vi "维持时间参数检查.vi"(7 "队列输入":refnum<queue>, 8 "NewVal输入":T1 {"时序参数"."nplc" min=0.001; "测试参数"."极限电流(mA)" min=0.0 max=3000.0; "测试参数"."读取电压(V)" min=0.0 max=40.0}, 11 "错误输入（无错误）":errorcluster) -> (0 "NewVal输出":T1 {"时序参数"."nplc" min=0.001; "测试参数"."极限电流(mA)" min=0.0 max=3000.0; "测试参数"."读取电压(V)" min=0.0 max=40.0}, 3 "错误输出":errorcluster)   [LabVIEW 2021]
uses:
  QueueLib/QueueLib.lvlib
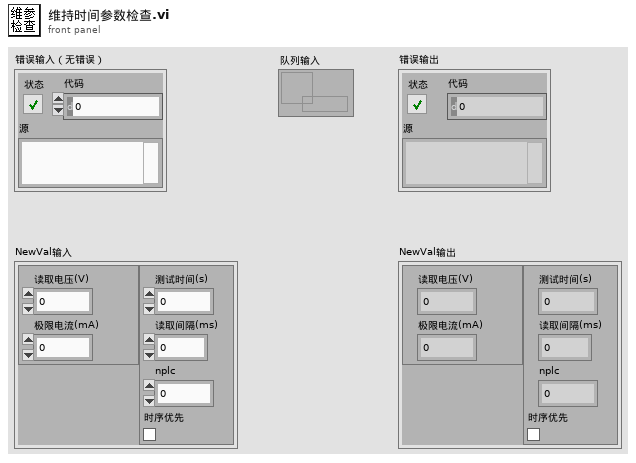
[diagram p1: front panel]
types:
  T1 = typedef "维持时间.ctl" = cluster{"测试参数":cluster{"读取电压(V)":dbl, "极限电流(mA)":dbl}, "时序参数":cluster{"测试时间(s)":dbl, "读取间隔(ms)":dbl, "nplc":dbl, "时序优先":bool}}
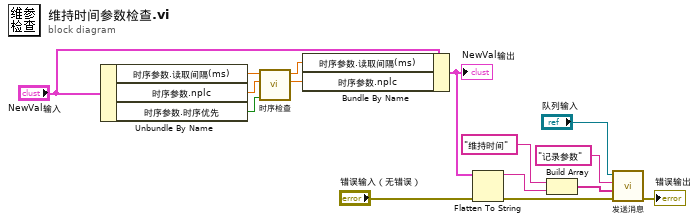
[diagram p0: block diagram]
diagram:
  n1 = Unbundle By Name("NewVal输入") -> ("时序参数.读取间隔(ms)"=w1:dbl, "时序参数.nplc"=w2:dbl, "时序参数.时序优先"=w3:bool)
  n2 = call "时序检查.vi"("时序优先"=w3, "nplc"=w2, "测量间隔"=w1) -> ("nplc输出"=w5:dbl, "测量间隔输出"=w4:dbl)  [unwired: 7 in]
  n3 = Bundle By Name(cluster="NewVal输入", "时序参数.读取间隔(ms)"=w4, "时序参数.nplc"=w5) -> (w15:T1)
  "NewVal输出" <- w15
  n4 = Flatten To String(anything=w15, error in (no error)="错误输入（无错误）") -> (data string=w8:string, error out=w6:errorcluster)  [unwired: 2 in, 1 out]
  n5 = Build Array("维持时间" ("元素"), w8) -> (w10:string[])
  n6 = call-poly "发送消息.vi"("错误输入（无错误）"=w6, "数据"=w10, "消息"="记录参数", "输入队列"="队列输入") -> ("错误输出"=→"错误输出":errorcluster)  [unwired: 6 in, 1 out]
